vi "Random1.vi"(1 "Random_num":dbl) -> (0 "배열":i32[](array[numeric]))   [LabVIEW 2014]
panel:
  out "난수(0에서 1)":dbl
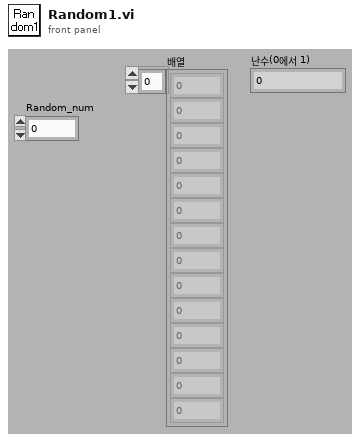
[diagram p1: front panel]
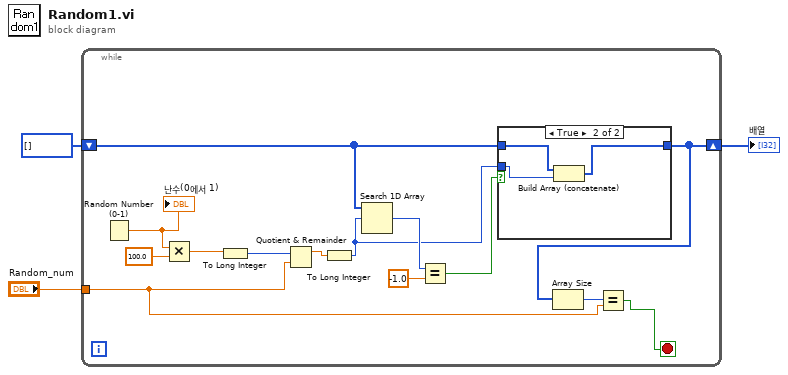
[diagram p0: block diagram]
diagram:
  n1 = while {
    tunnel: "Random_num" -> [w4]
    shift-right: [w7] -> w2
    shift-left: i32[] [] -> [w11]
    stop <- w5 stop-if-true
    n2 = Random Number (0-1)() -> (number: 0 to 1=w17:dbl)
    "난수(0에서 1)" <- w17
    n3 = Multiply(x=w17, y=100.0) -> (x*y=w15:dbl)
    n4 = To Long Integer(number=w15) -> (32bit integer=w10:i32)
    n5 = Quotient & Remainder(x=w10, y=w4) -> (x-y*floor(x/y)=w9:dbl)  [unwired: 1 out]
    n6 = To Long Integer(number=w9) -> (32bit integer=w8:i32)
    n7 = Search 1D Array(1D array=w11, element=w8) -> (index of element=w13:i32)  [unwired: 1 in]
    n8 = Equal?(x=w13, y=-1.0) -> (x = y?=w12:bool)
    n9 = case shown="True" w12 {
      tunnel: w8 -> [_ w21]
      tunnel: [w18 w20] -> w7
      tunnel: w11 -> [w18 w19]
      frame False {
      }
      frame True {
        n10 = Build Array (concatenate)(w19, w21) -> (w20:i32[])
      }
    }
    n11 = Array Size(array=w7) -> (size(s)=w6:i32)
    n12 = Equal?(x=w6, y=w4) -> (x = y?=w5:bool)
  }
  "배열" <- w2
